vi "fgv_Znorm_d4app.vi"(7 "Function":enum16{"Idle", "Write", "Read"}(ring), 8 "error in (no error)":errorcluster, 9 "Znorm_um_Scaling":dbl, 10 "acceptance angle":dbl, 11 "xyzNormalizedCoordinates":T1={"XYZ Start"=[{"X"=0.0, "Y"=0.0, "Z"=0.0}], "XYZ Stop"=[]}) -> (0 "error out":errorcluster, 2 "E Field":string[](array[string]), 3 "Phase Field":string[](array[string]))   [LabVIEW 2017]
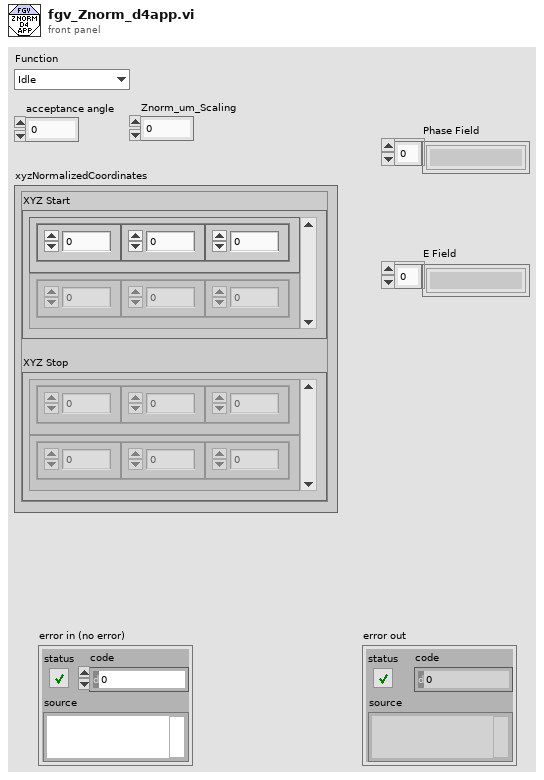
[diagram p1: front panel]
types:
  T1 = cluster{"XYZ Start":cluster{"X":sgl, "Y":sgl, "Z":sgl}[], "XYZ Stop":cluster{"X":sgl, "Y":sgl, "Z":sgl}[]}
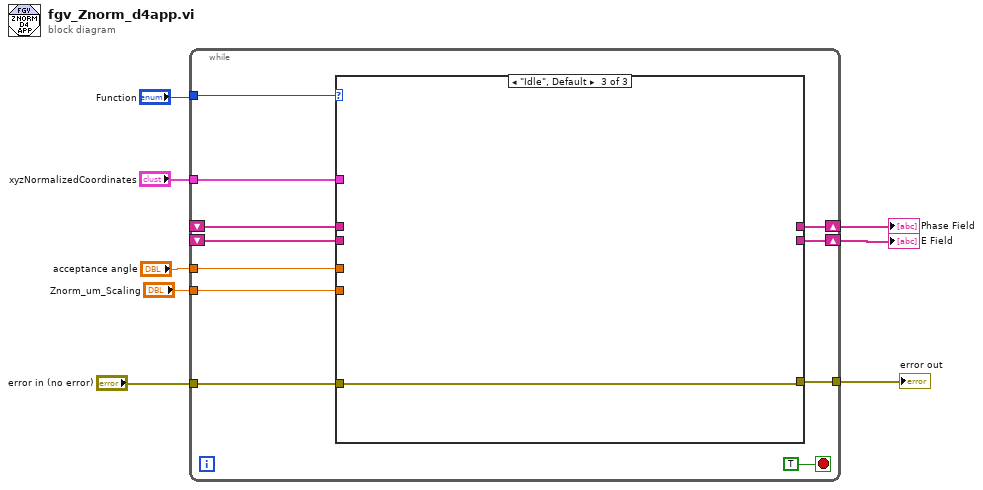
[diagram p0: block diagram]
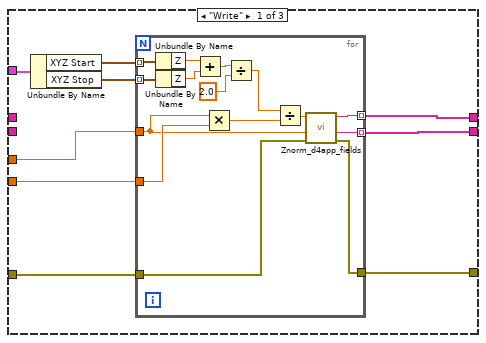
[diagram p2: hidden frame]
diagram:
  n1 = while {
    tunnel: "Function" -> [w18]
    shift-right: [w16] -> w7
    shift-left: _ -> [w17]
    shift-right: [w14] -> w6
    shift-left: _ -> [w15]
    tunnel: "xyzNormalizedCoordinates" -> [w13]
    tunnel: "acceptance angle" -> [w12]
    tunnel: "Znorm_um_Scaling" -> [w11]
    tunnel: "error in (no error)" -> [w10]
    tunnel: [w9] -> w1
    stop <- TRUE stop-if-true
    n2 = case shown="\"Idle\", Default" w18 {
      tunnel: w17 -> [_ w46 _]
      tunnel: [w27 w46 _] -> w16
      tunnel: w15 -> [_ w45 _]
      tunnel: [w28 w45 _] -> w14
      tunnel: w13 -> [w26 _ _]
      tunnel: w12 -> [w23 _ _]
      tunnel: w11 -> [w22 _ _]
      tunnel: w10 -> [w21 w44 w47]
      tunnel: [w20 w44 w47] -> w9
      frame "Write" {
        n3 = Unbundle By Name(w26) -> ("XYZ Start"=w25:cluster{"X":sgl, "Y":sgl, "Z":sgl}[], "XYZ Stop"=w24:cluster{"X":sgl, "Y":sgl, "Z":sgl}[])
        n4 = for {
          tunnel: [w43] -> w28 mode=indexing
          tunnel: [w42] -> w27 mode=indexing
          tunnel: w25 -> [w41] mode=indexing
          tunnel: w24 -> [w40] mode=indexing
          tunnel: w23 -> [w33]
          tunnel: w22 -> [w34]
          tunnel: w21 -> [w30]
          tunnel: [w29] -> w20
          n5 = Unbundle By Name(w41) -> ("Z"=w39:sgl)
          n6 = Unbundle By Name(w40) -> ("Z"=w38:sgl)
          n7 = Add(x=w39, y=w38) -> (x+y=w37:sgl)
          n8 = Multiply(x=w33, y=w34) -> (x*y=w32:dbl)
          n9 = Divide(x=w37, y=sgl 2.0) -> (x/y=w35:sgl)
          n10 = Divide(x=w35, y=w32) -> (x/y=w31:dbl)
          n11 = call "Znorm_d4app_fields.vi"("error in (no error)"=w30, "acceptance angle"=w33, "Zn"=w31) -> ("error out"=w29:errorcluster, "E field"=w43:string, "Phase Field"=w42:string)  [unwired: 6 in]
        }
      }
      frame "Read" {
      }
      frame "Idle", Default {
      }
    }
  }
  "E Field" <- w6
  "Phase Field" <- w7
  "error out" <- w1
